vi "Insert Cluster.vi"(8 "error in (no error)":errorcluster, 9 "Artist ID":i64, 10 "Name":string, 11 "SQLite Connection in":refnum<class "Connection.lvclass">) -> (0 "error out":errorcluster, 3 "SQLite Connection out":refnum<class "Connection.lvclass">)   [LabVIEW 2017]
doc: "Adds a new album to the database."
uses:
  <vilib>/drjdpowell/SQLite Library/SQL Connection/Connection.lvclass
  <vilib>/drjdpowell/SQLite Library/SQL Statement/SQL Statement.lvclass/SQL Statement.ctl
  <vilib>/drjdpowell/SQLite Library/SQL Statement/Bind Text.vi
  <vilib>/drjdpowell/SQLite Library/SQL Statement/Bind Integer.vi
  <vilib>/drjdpowell/SQLite Library/SQL Statement/Step.vi
  <vilib>/drjdpowell/SQLite Library/SQL Statement/Error Message.vi
  <vilib>/drjdpowell/SQLite Library/SQL Statement/SQL Statement.lvclass
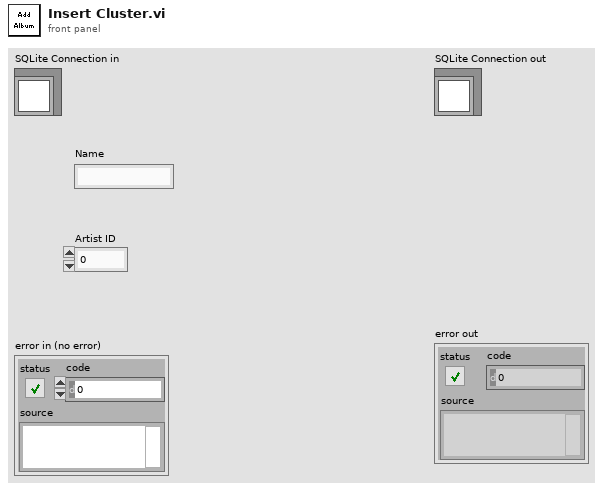
[diagram p1: front panel]
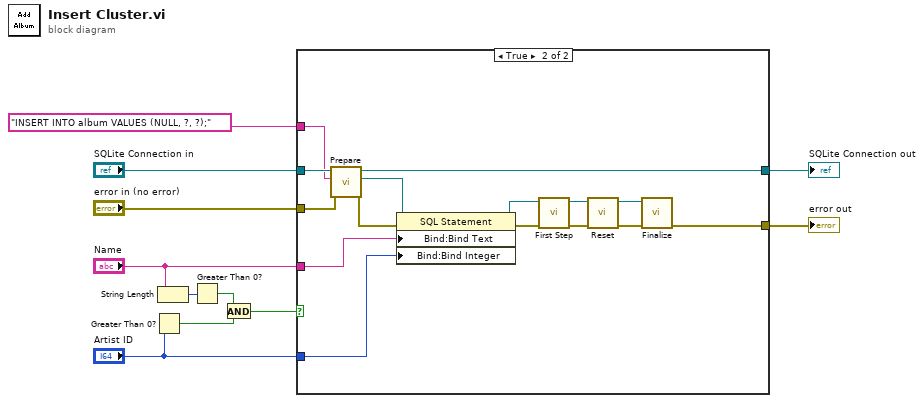
[diagram p0: block diagram]
diagram:
  n1 = Greater Than 0?(x="Artist ID") -> (x > 0?=w9:bool)
  n2 = String Length(string="Name") -> (length=w11:i32)
  n3 = Greater Than 0?(x=w11) -> (x > 0?=w10:bool)
  n4 = And(x=w10, y=w9) -> (x .and. y?=w8:bool)
  n5 = case shown="True" w8 {
    tunnel: "SQLite Connection in" -> [w13 w28]
    tunnel: "error in (no error)" -> [w12 w27]
    tunnel: "INSERT INTO album VALUES (NULL, ?, ?);" -> [_ w26]
    tunnel: "Name" -> [_ w23]
    tunnel: "Artist ID" -> [_ w22]
    tunnel: [w13 w15] -> w2
    tunnel: [w12 w14] -> w1
    frame False {
    }
    frame True {
      n6 = call <vilib>:"Prepare.vi"("error in (no error)"=w27, "SQL"=w26, "SQLite Connection in"=w28) -> ("error out"=w25:errorcluster, "SQL Statement"=w24:refnum<class "SQL Statement.lvclass">, "SQLite Connection"=w15:refnum<class "Connection.lvclass">)  [unwired: 4 in, 2 out]
      n7 = property class="SQL Statement"(reference=w24, error in=w25, "Bind:Bind Text"=w23, "Bind:Bind Integer"=w22) -> (reference out=w20:refnum<class "SQL Statement.lvclass">, error out=w21:errorcluster)
      n8 = call <vilib>:"First Step.vi"("error in (no error)"=w21, "SQL Statement in"=w20) -> ("error out"=w18:errorcluster, "SQL Statement"=w19:refnum<class "SQL Statement.lvclass">)  [unwired: 7 in, 1 out]
      n9 = call <vilib>:"Reset.vi"("error in (no error)"=w18, "SQL Statement in"=w19) -> ("error out"=w17:errorcluster, "SQL Statement"=w16:refnum<class "SQL Statement.lvclass">)  [unwired: 8 in]
      n10 = call <vilib>:"Finalize.vi"("error in (no error)"=w17, "SQL Statement in"=w16) -> ("error out"=w14:errorcluster)  [unwired: 9 in]
    }
  }
  "SQLite Connection out" <- w2
  "error out" <- w1
